vi "Calibrate Camera.vi"() -> ()   [LabVIEW 2020]
uses:
  g_ar_toolkit.ar/Camera Parameters.ctl
  g_ar_toolkit.ar/Camera Matrix.ctl
  g_ar_toolkit.ar/Camera Distortion Coefficients.ctl
  g_ar_toolkit.feature_detection/Chessboard Corner Info.ctl
  g_ar_toolkit.common/Object Point (Float).ctl
  g_ar_toolkit.image/ARGB Colour.ctl
  g_ar_toolkit.image/CreateEmptyImageGreyscale.vi
  g_ar_toolkit.image/ReadImageFileARGB.vi
  g_ar_toolkit.feature_detection/FindChessboardCornersGreyscale.vi
  g_ar_toolkit.image/GreyscaleImageSize.vi
  g_ar_toolkit.image/DrawArrowedLineOnImageARGB.vi
  g_ar_toolkit.image/DrawImageToPictureARGB.vi
  g_ar_toolkit.image/CreateEmptyImageGreyscale.vi/6598b9e0-8a08-46f5-91fd-ca1b87217137.vi
  g_ar_toolkit.image/CreateEmptyImageARGB.vi/3321fa97-f432-4e1e-8db9-a0df79aed21b.vi
  g_ar_toolkit.image/ReadImageFileARGB.vi/2358f293-6357-4b7a-bec3-c4e4d03be6e5.vi
  g_ar_toolkit.image/ARGBExtractChannel.vi
  g_ar_toolkit.feature_detection/FindChessboardCornersGreyscale.vi/ca99938f-1423-42fb-b653-ffd1f73e2bb5.vi
  g_ar_toolkit.image/GreyscaleImageSize.vi/69a1505b-b287-44ed-9ef9-f10ed7b260f4.vi
  g_ar_toolkit.image/DrawArrowedLineOnImageARGB.vi/c990ea83-8feb-41a3-987e-5529af170d73.vi
  g_ar_toolkit.image/DrawImageToPictureARGB.vi/8cd07b1b-062e-4fe4-9e87-2eb3dc89fe0e.vi
  <vilib>/Utility/error.llb/Error Cluster From Error Code.vi
  g_ar_toolkit.image/ARGBColourToU32.vi
  g_ar_toolkit.common/Termination Criteria/Get Values.vi
  g_ar_toolkit.common/Termination Criteria/Termination Criteria.lvclass
  g_ar_toolkit.image/CreateEmptyImageARGB.vi
  g_ar_toolkit.feature_detection/g_ar_toolkit.feature_detection.lvlib
  g_ar_toolkit.image/g_ar_toolkit.image.lvlib
  g_ar_toolkit.common/g_ar_toolkit.common.lvlib
  g_ar_toolkit.ar/g_ar_toolkit.ar.lvlib
panel:
  out "Results":picture[](array[picture])
  out "RMS Error":dbl[](array[numeric])
  out "Camera Parameters":T1
  # "This will be a low quality calibration because the calibration data set is too small and lacks variation"
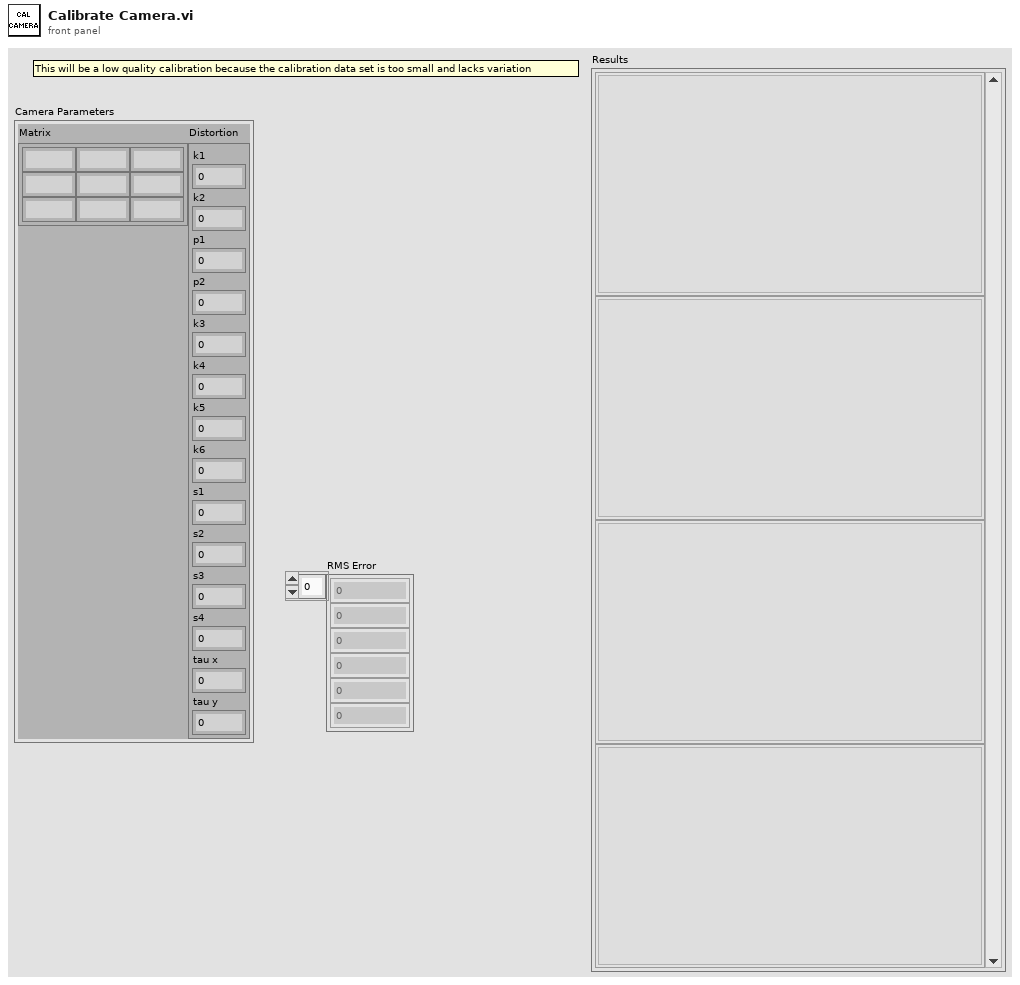
[diagram p1: front panel]
types:
  T1 = typedef "g_ar_toolkit.ar.lvlib/Camera Parameters.ctl" = cluster{"Matrix":T2, "Distortion":T3}
  T2 = typedef "g_ar_toolkit.ar.lvlib/Camera Matrix.ctl" = cluster{"m 0,0":dbl, "m 0,1":dbl, "m 0,2":dbl, "m 1,0":dbl, "m 1,1":dbl, "m 1,2":dbl, "m 2,0":dbl, "m 2,1":dbl, "m 2,2":dbl}
  T3 = typedef "g_ar_toolkit.ar.lvlib/Camera Distortion Coefficients.ctl" = cluster{"k1":dbl, "k2":dbl, "p1":dbl, "p2":dbl, "k3":dbl, "k4":dbl, "k5":dbl, "k6":dbl, "s1":dbl, "s2":dbl, "s3":dbl, "s4":dbl, "tau x":dbl, "tau y":dbl}
  T4 = typedef "g_ar_toolkit.image.lvlib/ARGB Colour.ctl" = cluster{"Alpha":u8, "RGB":u32}
  T5 = typedef "g_ar_toolkit.common.lvlib/Object Point (Float).ctl" = cluster{"x":dbl, "y":dbl, "z":dbl}
  T6 = typedef "g_ar_toolkit.feature_detection.lvlib/Chessboard Corner Info.ctl" = cluster{"Points Per Row":u8, "Points Per Col":u8}
  T7 = cluster{"Points Per Row":i32, "Points Per Col":i32}
  T8 = typedef "g_ar_toolkit.common.lvlib/Image Point (Float).ctl" = cluster{"x":dbl, "y":dbl}
  T9 = typedef "g_ar_toolkit.common.lvlib/Image Size (Integer).ctl" = cluster{"Width":u16, "Height":u16}
  T10 = typedef "g_ar_toolkit.ar.lvlib/Pose.ctl" = cluster{"rvec":T11, "tvec":T12}
  T11 = typedef "g_ar_toolkit.ar.lvlib/rvec.ctl" = cluster{"v0":dbl, "v1":dbl, "v2":dbl}
  T12 = typedef "g_ar_toolkit.ar.lvlib/tvec.ctl" = cluster{"x":dbl, "y":dbl, "z":dbl}
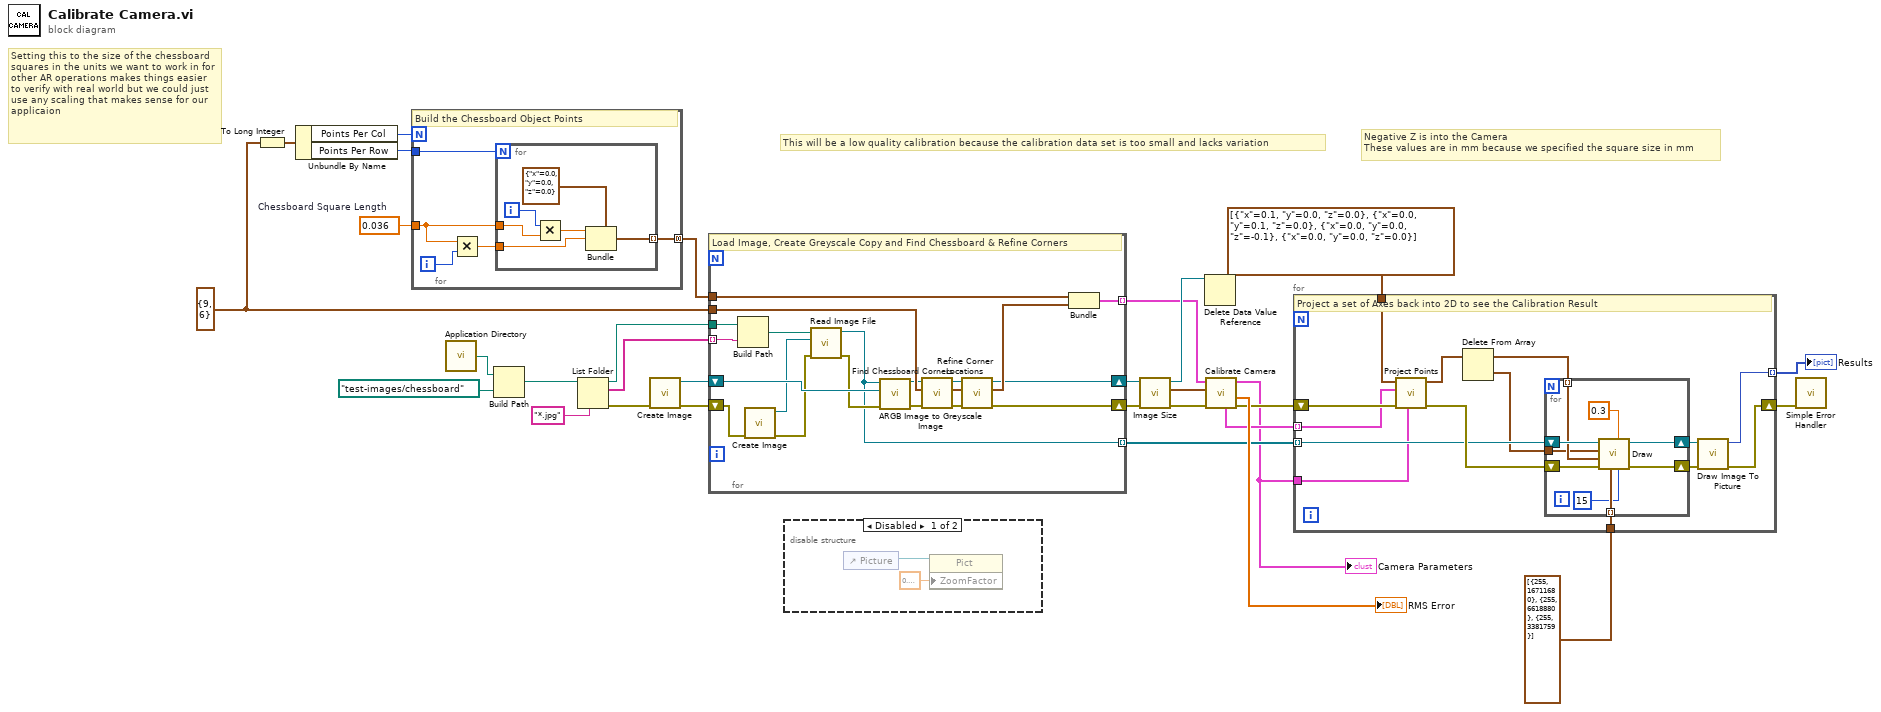
[diagram p0: block diagram]
diagram:
  w10 = 0.036  # Chessboard Square Length
  w21 = T6 {"Points Per Row"=9, "Points Per Col"=6} ("Chessboard Corners Info")
  # "Setting this to the size of the chessboard squares in the units we want to work in for other AR operations makes things easier to verify with real world but we could just use any scaling that makes sense for our applicaion"
  # "Negative Z is into the Camera\nThese values are in mm because we specified the square size in mm"
  # "This will be a low quality calibration because the calibration data set is too small and lacks variation"
  n1 = To Long Integer(number=w21) -> (32bit integer=w17:T7)
  n2 = Unbundle By Name(w17) -> ("Points Per Col"=w20:i32, "Points Per Row"=w19:i32)
  n3 = for {
    N: w20 -> [_]
    tunnel: w19 -> [w35]
    tunnel: w10 -> [w33]
    tunnel: [w31] -> w18 mode=concatenating
    i -> [w34]
    # "Build the Chessboard Object Points"
    n4 = Multiply(x=w33, y=w34) -> (x*y=w32:dbl)
    n5 = for {
      N: w35 -> [_]
      tunnel: w33 -> [w41]
      tunnel: w32 -> [w37]
      tunnel: [w36] -> w31 mode=indexing
      i -> [w40]
      n6 = Multiply(x=w40, y=w41) -> (x*y=w38:dbl)
      n7 = Bundle(cluster=T5 {"x"=0.0, "y"=0.0, "z"=0.0} ("Object Point"), "x"=w38, "y"=w37) -> (w36:T5)  [unwired: 1 in]
    }
  }
  n8 = call <vilib>:"Application Directory.vi"() -> ("Application Directory"=w27:path)
  n9 = Build Path(base path=w27, name or relative path=path "test-images/chessboard") -> (appended path=w25:path)
  n10 = List Folder(path=w25, pattern="*.jpg") -> (path out=w24:path, filenames=w22:string[], error out=w23:errorcluster)  [unwired: 2 in, 1 out]
  n11 = call-poly "Create Image.vi"("error in (no error)"=w23) -> ("error out"=w29:errorcluster, "New Greyscale Image"=w30:refnum<data-value>)  [unwired: 9 in]
  n12 = for {
    tunnel: w24 -> [w61]
    tunnel: w22 -> [w60] mode=indexing
    shift-right: [w58] -> w13
    shift-left: w29 -> [w46]
    shift-right: [w51] -> w15
    shift-left: w30 -> [w50]
    tunnel: w21 -> [w57]
    tunnel: w18 -> [w56]
    tunnel: [w55] -> w2 mode=indexing
    tunnel: [w42] -> w8 mode=indexing
    # "Load Image, Create Greyscale Copy and Find Chessboard & Refine Corners"
    n13 = Build Path(base path=w61, name or relative path=w60) -> (appended path=w59:path)
    n14 = call-poly "Create Image.vi"("error in (no error)"=w46) -> ("error out"=w45:errorcluster, "New ARGB Image"=w44:refnum<data-value>)  [unwired: 9 in]
    n15 = call-poly "Read Image File.vi"("error in (no error)"=w45, "ARGB Image Destination"=w44, "Filepath"=w59) -> ("error out"=w43:errorcluster, "ARGB Image Destination (duplicate)"=w42:refnum<data-value>)  [unwired: 7 in]
    n16 = call "ARGB Image to Greyscale Image.vi"("error in (no error)"=w43, "Greyscale Image Destination"=w50, "ARGB Image Source"=w42) -> ("error out"=w47:errorcluster, "Greyscale Image Destination (Duplicate)"=w49:refnum<data-value>)  [unwired: 7 in]
    n17 = call-poly "Find Chessboard Corners.vi"("error in (no error)"=w47, "Chessboard Corners Info"=w57, "Greyscale Image"=w49) -> ("error out"=w54:errorcluster, "Points"=w53:T8[], "Greyscale Image (Duplicate)"=w48:refnum<data-value>)  [unwired: 6 in]
    n18 = call "Refine Corner Locations.vi"("error in (no error)"=w54, "Points in"=w53, "Greyscale Image"=w48) -> ("error out"=w58:errorcluster, "Points out"=w52:T8[], "Greyscale Image (Duplicate)"=w51:refnum<data-value>)  [unwired: 6 in]
    n19 = Bundle(w56, "Points out"=w52) -> (w55:cluster{T5[], "Points out":T8[]})  [unwired: 1 in]
  }
  n20 = disable-structure shown="Disabled" {
    frame Disabled {
      n21 = control-ref of="Picture"() -> (w63:refnum<vi>)
      n22 = property class="Pict"(reference=w63, "ZoomFactor"=sgl 0.2 ("Zoom Factor")) -> ()  [unwired: 1 in, 2 out]
    }
    frame Enabled {
    }
  }
  n23 = call-poly "Image Size.vi"("error in (no error)"=w13, "Greyscale Image"=w15) -> ("error out"=w12:errorcluster, "Image Size"=w11:T9, "Greyscale Image (duplicate)"=w14:refnum<data-value>)  [unwired: 7 in]
  n24 = Delete Data Value Reference(data value reference=w14) -> ()  [unwired: 1 in, 2 out]
  n25 = call "Calibrate Camera.vi"("error in (no error)"=w12, "Image Size"=w11, "Point Correspondences"=w2) -> ("error out"=w7:errorcluster, "RMS Error"=→"RMS Error":dbl[], "Camera Parameters"=w6:T1, "Poses"=w9:T10[])  [unwired: 5 in]
  "Camera Parameters" <- w6
  n26 = for {
    tunnel: w9 -> [w64] mode=indexing
    tunnel: w8 -> [w75] mode=indexing
    shift-right: [w69] -> w1
    shift-left: w7 -> [w65]
    tunnel: w6 -> [w66]
    tunnel: T5[] [{"x"=0.1, "y"=0.0, "z"=0.0}, {"x"=0.0, "y"=0.1, "z"=0.0}, {"x"=0.0, "y"=0.0, "z"=-0.1}, {"x"=0.0, "y"=0.0, "z"=0.0}] ("Object Points") -> [w77]
    tunnel: T4[] [{"Alpha"=255, "RGB"=16711680}, {"Alpha"=255, "RGB"=6618880}, {"Alpha"=255, "RGB"=3381759}] -> [w71]
    tunnel: [w67] -> w3 mode=indexing
    # "Project a set of Axes back into 2D to see the Calibration Result"
    n27 = call "Project Points.vi"("Camera Parameters"=w66, "error in (no error)"=w65, "Pose"=w64, "Object Points"=w77) -> ("error out"=w76:errorcluster, "Image Points"=w74:T8[])  [unwired: 6 in]
    n28 = Delete From Array(array=w74) -> (deleted portion=w73:T8, array with subset deleted=w72:T8[])  [unwired: 2 in]
    n29 = for {
      shift-right: [w83] -> w68
      shift-left: w75 -> [w84]
      tunnel: w73 -> [w78]
      tunnel: w72 -> [w79] mode=indexing
      tunnel: w71 -> [w82] mode=indexing
      shift-right: [w81] -> w70
      shift-left: w76 -> [w86]
      n30 = call-poly "Draw.vi"("Thickness (Default: 1)"=15, "Tip Length (Default 0.1)"=0.3, "ARGB Colour"=w82, "error in (no error)"=w86, "Pointed-to Point"=w79, "Start Point"=w78, "ARGB Image"=w84) -> ("error out"=w81:errorcluster, "ARGB Image (Duplicate)"=w83:refnum<data-value>)  [unwired: 3 in]
    }
    n31 = call-poly "Draw Image To Picture.vi"("error in (no error)"=w70, "ARGB Image Source"=w68) -> ("error out"=w69:errorcluster, "Picture"=w67:picture)  [unwired: 8 in]
  }
  "Results" <- w3
  n32 = call <vilib>:"Simple Error Handler.vi"("error in (no error)"=w1) -> ()  [unwired: 4 in, 5 out]
